vi "DH - Define home.vi"(1 "Axis":i8=1 min=1 max=6 step=1, 2 "error in":errorcluster, 3 "Set this # as the\nhome - default is 0.00":dbl format="%.2f", 4 "Address / Port":i16=1 min=1 max=31 step=1) -> (0 "error out":errorcluster)   [LabVIEW 2014]
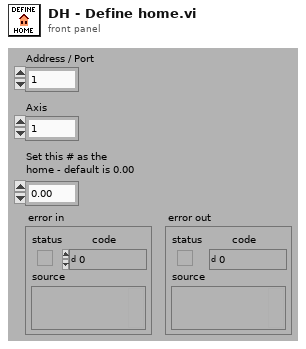
[diagram p1: front panel]
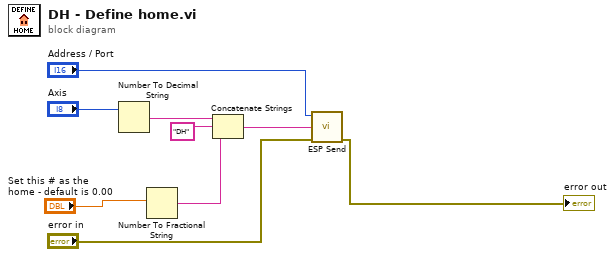
[diagram p0: block diagram]
diagram:
  n1 = Number To Decimal String(number="Axis") -> (decimal integer string=w8:string)  [unwired: 1 in]
  n2 = Number To Fractional String(number="Set this # as the\nhome - default is 0.00") -> (F-format string=w5:string)  [unwired: 3 in]
  n3 = Concatenate Strings(w8, "DH" ("Substring"), w5) -> (w2:string)
  n4 = call "ESP Send.vi"("error in"="error in", "Command String"=w2, "Address / Port"="Address / Port") -> ("error out"=→"error out":errorcluster)  [unwired: 3 in, 1 out]
